vi "getNodePrototypes.vi"(0 "reference":refnum<class "Graph.lvclass">, 1 "NodeName":string, 5 "error in (no error)":errorcluster) -> (14 "reference out":refnum<class "Graph.lvclass">, 15 "nodes":refnum<class "AbstractNode.lvclass">[](array[class]), 16 "node":refnum<class "AbstractNode.lvclass">, 19 "error out":errorcluster)   [LabVIEW 2014, in "Graph.lvclass"]
uses:
  <resource>/Framework/Providers/Open_GDS/UML/Graph_class/Graph.lvclass
  <resource>/Framework/Providers/Open_GDS/UML/AbstractNode_class/AbstractNode.lvclass
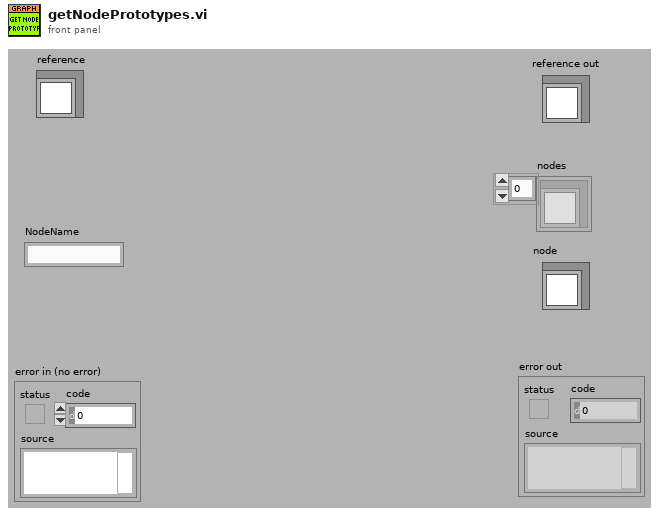
[diagram p1: front panel]
types:
  T1 = typedef "Graph.lvclass/ClassAttributes.ctl" = cluster{"NODE_PROT":refnum<class "AbstractNode.lvclass">[], "NodeNames":string[], "EDGE_PROT":refnum<class "AbstractEdge.lvclass">[], "EdgeNames":string[]}
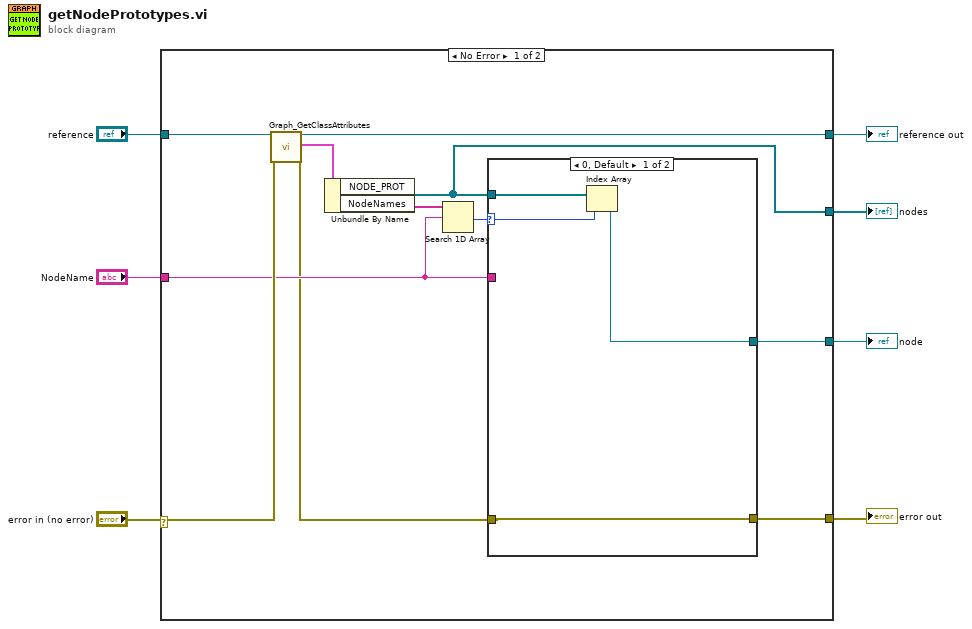
[diagram p0: block diagram]
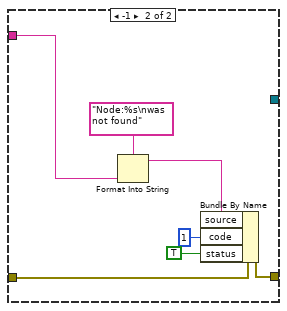
[diagram p2: hidden frame]
diagram:
  n1 = case shown="No Error" "error in (no error)" {
    selector: "error in (no error)" -> [w15 w29]
    tunnel: "reference" -> [w17 w30]
    tunnel: [w16 w29] -> w6
    tunnel: [w17 w30] -> w5
    tunnel: [w14 _] -> w3
    tunnel: "NodeName" -> [w13 _]
    tunnel: [w12 _] -> w1
    frame No Error {
      n2 = call <resource>:"Graph_GetClassAttributes.vi"("reference in"=w17, "error in (no error)"=w15) -> ("Class attribute"=w8:T1, "error out"=w9:errorcluster)  [unwired: 16 out]
      n3 = Unbundle By Name(w8) -> ("NODE_PROT"=w14:refnum<class "AbstractNode.lvclass">[], "NodeNames"=w11:string[])
      n4 = Search 1D Array(1D array=w11, element=w13) -> (index of element=w10:i32)  [unwired: 1 out]
      n5 = case shown="0, Default" w10 {
        selector: w10 -> [w20 _]
        tunnel: w13 -> [_ w27]
        tunnel: w9 -> [w18 w26]
        tunnel: [w18 w22] -> w16
        tunnel: w14 -> [w21 _]
        tunnel: [w19 _] -> w12
        frame 0, Default {
          n6 = Index Array(array=w21, index=w20) -> (element=w19:refnum<class "AbstractNode.lvclass">)
        }
        frame -1 {
          n7 = Format Into String(format string="Node:%s\nwas not found", w27) -> (resulting string=w24:string)  [unwired: 2 in, 1 out]
          n8 = Bundle By Name(cluster=w26, "source"=w24, "code"=1, "status"=TRUE) -> (w22:errorcluster)
        }
      }
    }
    frame Error {
    }
  }
  "reference out" <- w5
  "error out" <- w6
  "nodes" <- w3
  "node" <- w1
